vi "Client Complete Streaming Call.vi"(8 "error in":errorcluster, 11 "Call Id":T2) -> (0 "error out":errorcluster, 1 "errorDetails":T1)   [LabVIEW 2019, in "gprc-lvsupport.lvlib"]
uses:
  gprc-lvsupport.lvlib
  Shared/grpcId.ctl
  Shared/Any.ctl
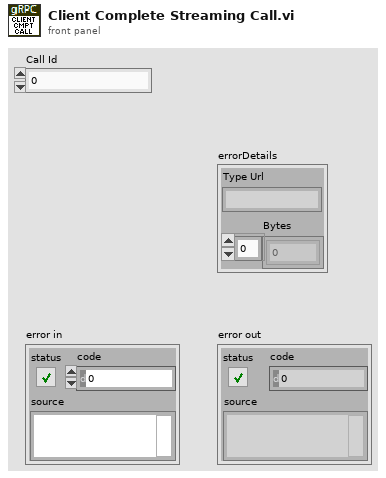
[diagram p1: front panel]
types:
  T1 = typedef "gprc-lvsupport.lvlib/Any.ctl" = cluster{"Type Url":string, "Bytes":u8[]}
  T2 = typedef "gprc-lvsupport.lvlib/grpcId.ctl" = u64
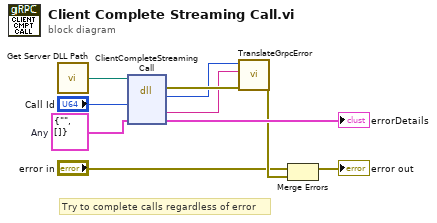
[diagram p0: block diagram]
diagram:
  w7 = T1 {"Type Url"="", "Bytes"=[]}  # Any
  # "Try to complete calls regardless of error"
  n1 = call "Get Server DLL Path.vi"() -> ("Server dll path"=w8:path)
  n2 = dll-call lib="?" fn="ClientCompleteStreamingCall"(path in=w8, "ClientId"="Call Id", "errorDetails"=w7) -> (error out=w10:errorcluster, "return type"=w4:i32, "errorMessage"=w5:string, "errorDetails"=→"errorDetails":T1)  [unwired: 4 in, 1 out]
  n3 = call "TranslateGrpcError.vi"("error in"=w10, "Error Message"=w5, "Error Code"=w4) -> ("error out"=w3:errorcluster)  [unwired: 8 in]
  n4 = Merge Errors("error in", w3) -> (→"error out":errorcluster)
